vi "test_TxUDP-RxUDP - Multiple Boards - 16 Channels.vi"(8 "error in":errorcluster, 11 "reference in":refnum<class "AIM ARINC 664 Loopback-MultiDevice.lvclass">) -> (0 "error out":errorcluster, 3 "reference out":refnum<class "AIM ARINC 664 Loopback-MultiDevice.lvclass">)   [LabVIEW 2020, in "AIM ARINC 664 Loopback-MultiDevice.lvclass"]
uses:
  AIM ARINC 664 Loopback-MultiDevice.lvclass
  C:/Program Files/National Instruments/LabVIEW 2024/vi.lib/NI/VeriStand Custom Device Testing Tools/VeriStandTestCase/VeriStandTestCase.lvclass
  AIM ARINC 664 Loopback-MultiDevice.lvclass/AIM ARINC 664 Loopback-MultiDevice.ctl
  b47c41b5-a02e-49d5-b852-4e28f097d7ad.vi
  6a3dd3ed-914d-4d14-bf18-724521aa5e28.vi
  8abe1e9f-12f7-4d29-bb0e-ea5e1950c3f4.vi
  NationalInstruments.VeriStand.SystemDefinitionAPI
  <vilib>/addons/_JKI Toolkits/VI Tester/TestCase.llb/TestCase.lvclass
  Scripting/AIM ARINC 664 Scripting.lvlib
  <vilib>/NI/VeriStand Custom Device Testing Tools/VeriStandTestCase/VeriStandTestCase.lvclass
  C:/Program Files/National Instruments/LabVIEW 2024/vi.lib/addons/_JKI Toolkits/VI Tester/TestCase.llb/TestCase.lvclass
panel:
  in  "# of channels":i32=16
  out "resulting string":string
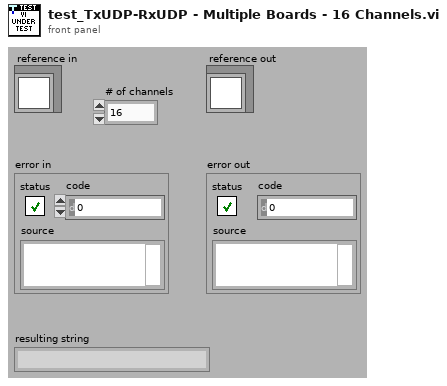
[diagram p1: front panel]
types:
  T1 = typedef "Custom Device API.lvlib/Custom Device Item Ref.ctl" = u64
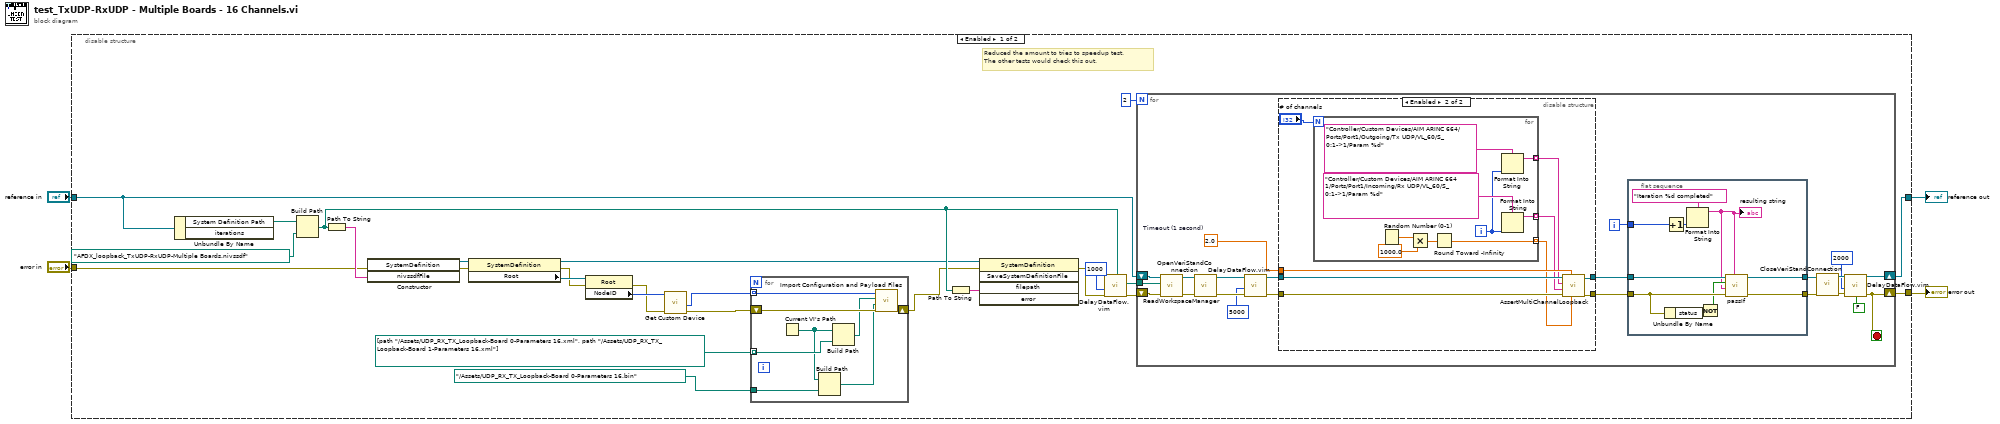
[diagram p0: block diagram]
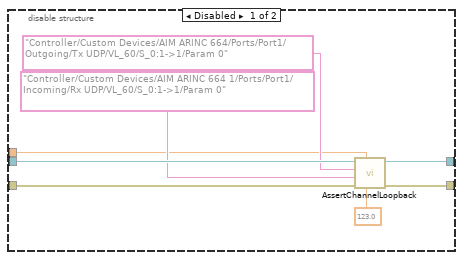
[diagram p2: hidden frame]
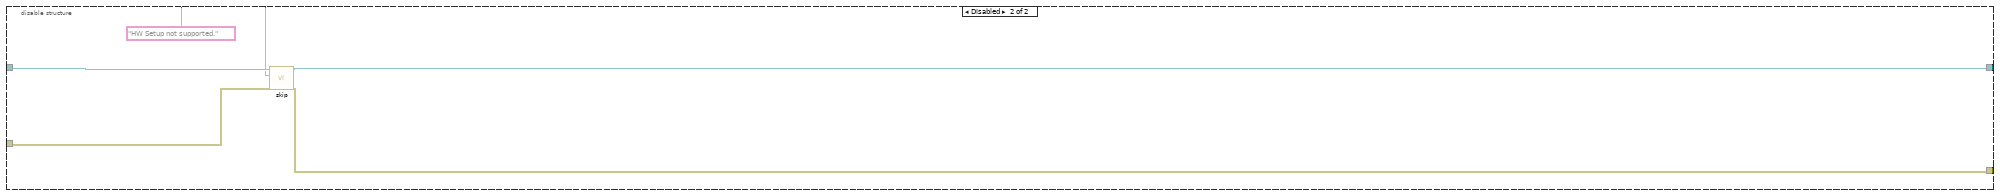
[diagram p3: hidden frame]
diagram:
  n1 = disable-structure shown="Enabled" {
    disable-tunnel: "reference in" -> [w10 w98]
    disable-tunnel: "error in" -> [w9 w97]
    disable-tunnel: [w27 w96] -> w2
    disable-tunnel: [w26 w95] -> w1
    frame Enabled {
      # "Reduced the amount to tries to speedup test.\nThe other tests would check this out."
      n2 = Unbundle By Name(w10) -> ("System Definition Path"=w29:path)  [unwired: 1 out]
      n3 = Build Path(base path=w29, name or relative path=path "AFDX_loopback_TxUDP-RxUDP-Multiple Boards.nivssdf") -> (appended path=w24:path)
      n4 = Path To String(path=w24) -> (string=w25:string)
      n5 = constructor class="SystemDefinition"(error in=w9, "nivssdfFile"=w25) -> (reference out=w23:refnum<k24>, error out=w21:errorcluster)  [unwired: 2 in, 2 out]
      n6 = property class="SystemDefinition"(reference=w23, error in=w21) -> (reference out=w18:refnum<k24>, error out=w20:errorcluster, "Root"=w22:refnum<k24>)
      n7 = property class="Root"(reference=w22, error in=w20) -> (error out=w15:errorcluster, "NodeID"=w16:u64)  [unwired: 1 out]
      n8 = call "Get Custom Device.vi"("error in"=w15, "custom device ref in"=w16) -> ("error out"=w14:errorcluster, "Item Refs"=w8:T1[])  [unwired: 5 in, 3 out]
      n9 = for {
        shift-right: [w36] -> w19
        shift-left: w14 -> [w37]
        tunnel: path[] [path "../Assets/UDP_RX_TX_Loopback-Board 0-Parameters 16.xml", path "../Assets/UDP_RX_TX_Loopback-Board 1-Parameters 16.xml"] -> [w33] mode=indexing
        tunnel: w8 -> [w32] mode=indexing
        tunnel: path "../Assets/UDP_RX_TX_Loopback-Board 0-Parameters 16.bin" -> [w30]
        n10 = Current VI's Path() -> (path=w31:path)
        n11 = Build Path(base path=w31, name or relative path=w30) -> (appended path=w35:path)
        n12 = Build Path(base path=w31, name or relative path=w33) -> (appended path=w34:path)
        n13 = call "Import Configuration and Payload Files.vi"("error in"=w37, "payload file path"=w35, "parameters configuration file path"=w34, "custom device ref"=w32) -> ("error out"=w36:errorcluster)  [unwired: 6 in, 1 out]
      }
      n14 = Path To String(path=w24) -> (string=w17:string)
      n15 = invoke class="SystemDefinition" method="SaveSystemDefinitionFile"(reference=w18, error in=w19, "filepath"=w17) -> (error out=w13:errorcluster)  [unwired: 2 in, 4 out]
      n16 = call "DelayDataFlow.vim"("value in"=w13, "milliseconds to wait"=u32 1000) -> ("value out"=w12:errorcluster)  [unwired: 2 in, 1 out]
      n17 = for {
        N: 2 -> [_]
        tunnel: w24 -> [w50]
        shift-right: [w55] -> w26
        shift-left: w10 -> [w57]
        shift-right: [w39] -> w27
        shift-left: w12 -> [w51]
        i -> [w41]
        stop <- w39 stop-if-true
        w38 = 2.0  # Timeout (1 second)
        n18 = call-dynamic "OpenVeriStandConnection.vi"("error in (no error)"=w51, "System Definition File"=w50, "VeriStand Test Case in"=w57) -> ("error out"=w56:errorcluster, "VeriStand Test Case out"=w54:refnum<class "AIM ARINC 664 Loopback-MultiDevice.lvclass">)  [unwired: 6 in, 1 out]
        n19 = call-dynamic "ReadWorkspaceManager.vi"("error in (no error)"=w56, "VeriStand Test Case in"=w54) -> ("error out"=w53:errorcluster, "VeriStand Test Case out"=w48:refnum<class "AIM ARINC 664 Loopback-MultiDevice.lvclass">)  [unwired: 7 in, 1 out]
        n20 = call "DelayDataFlow.vim"("value in"=w53, "milliseconds to wait"=u32 5000) -> ("value out"=w49:errorcluster)  [unwired: 2 in, 1 out]
        n21 = disable-structure shown="Enabled" {
          disable-tunnel: w49 -> [w65 w71]
          disable-tunnel: w48 -> [w64 w74]
          disable-tunnel: [w62 w72] -> w42
          disable-tunnel: [w61 w73] -> w40
          disable-tunnel: w38 -> [w58 w70]
          frame Disabled {
            n22 = call <vilib>:"AssertChannelLoopback.vi"("Value"=123.0, "Timeout (1 second)"=w58, "error in (no error)"=w65, "Read Channel"="Controller/Custom Devices/AIM ARINC 664 1/Ports/Port1/Incoming/Rx UDP/VL_60/S_0:1->1/Param 0", "Write Channel"="Controller/Custom Devices/AIM ARINC 664/Ports/Port1/Outgoing/Tx UDP/VL_60/S_0:1->1/Param 0", "VeriStand Test Case in"=w64) -> ("error out"=w62:errorcluster, "VeriStand Test Case out"=w61:refnum<class "AIM ARINC 664 Loopback-MultiDevice.lvclass">)  [unwired: 4 in]
          }
          frame Enabled {
            n23 = for {
              N: "# of channels" -> [_]
              tunnel: [w80] -> w68 mode=indexing
              tunnel: [w76] -> w67 mode=indexing
              tunnel: [w75] -> w66 mode=indexing
              i -> [w77]
              n24 = Random Number (0-1)() -> (number: 0 to 1=w83:dbl)
              n25 = Multiply(x=w83, y=1000.0) -> (x*y=w81:dbl)
              n26 = Round Toward -Infinity(1:w81) -> (0:w80:dbl)
              n27 = Format Into String(format string="Controller/Custom Devices/AIM ARINC 664/Ports/Port1/Outgoing/Tx UDP/VL_60/S_0:1->1/Param %d", w77) -> (resulting string=w76:string)  [unwired: 2 in, 1 out]
              n28 = Format Into String(format string="Controller/Custom Devices/AIM ARINC 664 1/Ports/Port1/Incoming/Rx UDP/VL_60/S_0:1->1/Param %d", w77) -> (resulting string=w75:string)  [unwired: 2 in, 1 out]
            }
            n29 = call <vilib>:"AssertMultiChannelLoopback.vi"("Values"=w68, "Timeout (1 second)"=w70, "error in (no error)"=w71, "Read Channels"=w66, "Write Channels"=w67, "VeriStand Test Case in"=w74) -> ("error out"=w72:errorcluster, "VeriStand Test Case out"=w73:refnum<class "AIM ARINC 664 Loopback-MultiDevice.lvclass">)  [unwired: 4 in]
          }
        }
        n30 = flat-sequence {
          tunnel: [w93] -> w44
          tunnel: [w92] -> w43
          tunnel: w42 -> [w91]
          tunnel: w41 -> [w87]
          tunnel: w40 -> [w85]
          frame #0 {
            n31 = Unbundle By Name(w91) -> ("status"=w90:bool)
            n32 = Increment(x=w87) -> (x+1=w86:i32)
            n33 = Format Into String(format string="Iteration %d completed", w86) -> (resulting string=w84:string)  [unwired: 2 in, 1 out]
            "resulting string" <- w84
            n34 = Not(x=w90) -> (.not. x?=w89:bool)
            n35 = call-dynamic "passIf.vi"("custom report message (\"\")"=w84, "error in (no error)"=w91, "message (\"\")"=w84, "pass"=w89, "TestCase in"=w85) -> ("error out"=w92:errorcluster, "TestCase out"=w93:refnum<class "AIM ARINC 664 Loopback-MultiDevice.lvclass">)  [unwired: 5 in]
          }
        }
        n36 = call-dynamic "CloseVeriStandConnection.vi"("error in (no error)"=w43, "VeriStand Test Case in"=w44) -> ("error out"=w47:errorcluster, "VeriStand Test Case out"=w55:refnum<class "AIM ARINC 664 Loopback-MultiDevice.lvclass">)  [unwired: 8 in]
        n37 = call "DelayDataFlow.vim"("value in"=w47, "milliseconds to wait"=u32 2000, "no delay on error (T)"=FALSE) -> ("value out"=w39:errorcluster)  [unwired: 1 in, 1 out]
      }
    }
    frame Disabled {
      n38 = call <vilib>:"skip.vi"("error in (no error)"=w97, "skipMessage"="HW Setup not supported.", "TestCase in"=w98) -> ("error out"=w96:errorcluster, "TestCase out"=w95:refnum<class "AIM ARINC 664 Loopback-MultiDevice.lvclass">)  [unwired: 7 in]
    }
  }
  "error out" <- w2
  "reference out" <- w1
